vi "frontPanel.vi"(8 "error in (no error)":errorcluster, 10 "closeViewerEvent":refnum<user-event>, 11 "AnalysisResultsViewer in":refnum<class "AnalysisResultsViewer.lvclass">) -> (0 "error out":errorcluster, 3 "AnalysisResultsViewer out":refnum<class "AnalysisResultsViewer.lvclass">)   [LabVIEW 2011, in "Views.lvlib" / "Camera.lvlib" / "AnalysisResultsViewer.lvclass"]
uses:
  AnalysisResultsViewer.lvclass
  AnalysisResultsViewer.lvclass/AnalysisResultsViewer.ctl
panel:
  in  "timescale":dbl=1000.0
  in  "ResultsBox":i32(listbox)
  out "Cloud Size y":dbl(graph)
  in  "stop":bool
  out "Cloud Size x":dbl(graph)
  out "Atom Number":dbl(graph)
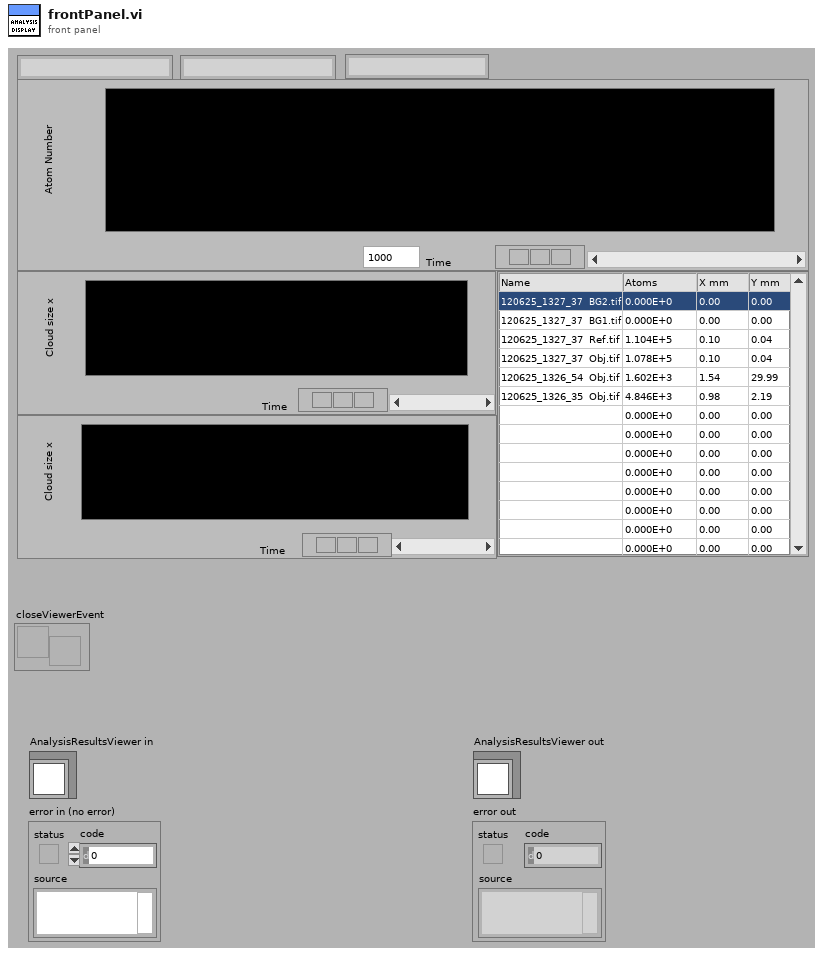
[diagram p1: front panel]
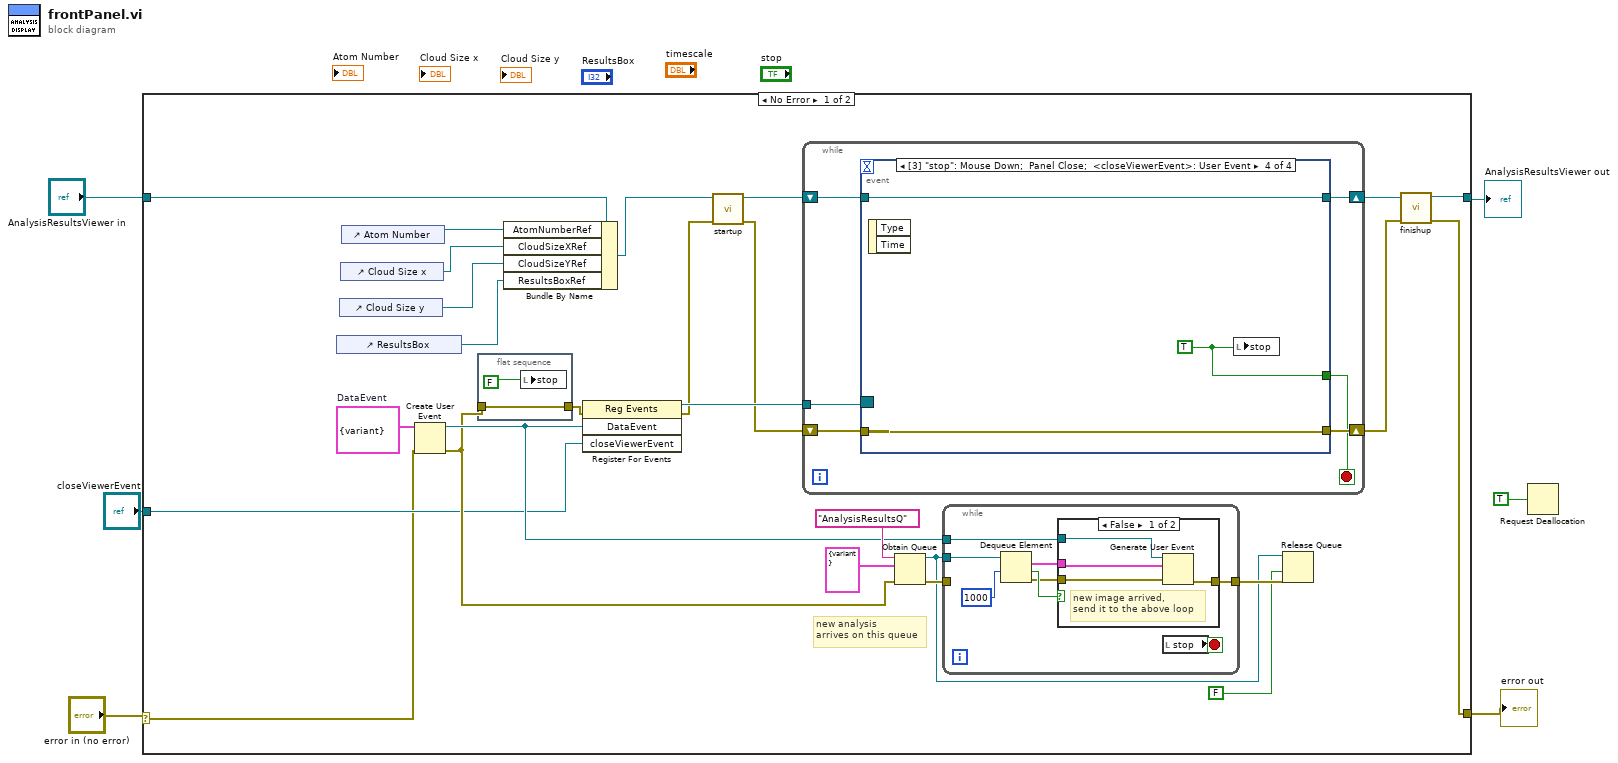
[diagram p0: block diagram]
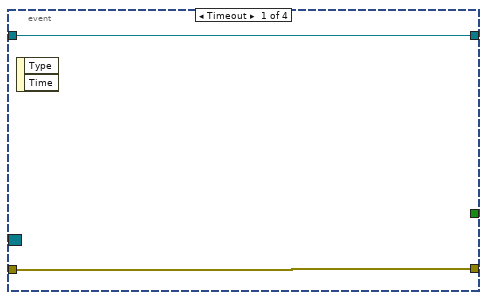
[diagram p3: hidden frame]
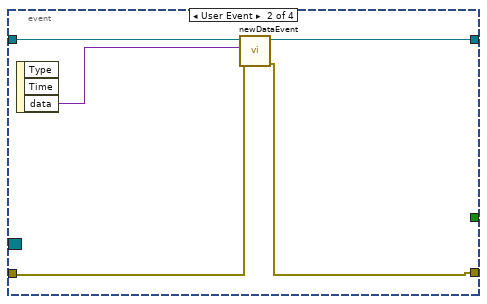
[diagram p4: hidden frame]
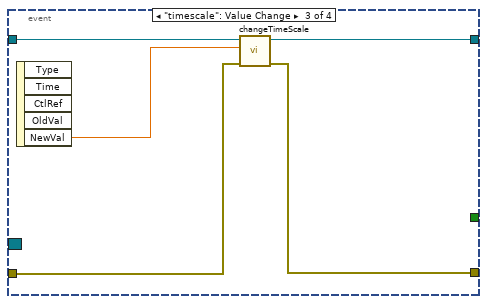
[diagram p5: hidden frame]
diagram:
  n1 = case shown="No Error" "error in (no error)" {
    selector: "error in (no error)" -> [w7 w70]
    tunnel: [w10 w70] -> w5
    tunnel: [w12 w69] -> w3
    tunnel: "AnalysisResultsViewer in" -> [w25 w69]
    tunnel: "closeViewerEvent" -> [w8 _]
    frame No Error {
      w27 = cluster{"data":variant} {"data"=variant}  # DataEvent
      # "new analysis\narrives on this queue"
      n2 = control-ref of="ResultsBox"() -> (w9:refnum<vi>)
      n3 = control-ref of="Cloud Size y"() -> (w22:refnum<vi>)
      n4 = control-ref of="Cloud Size x"() -> (w23:refnum<vi>)
      n5 = control-ref of="Atom Number"() -> (w24:refnum<vi>)
      n6 = Create User Event(user event datatype=w27, error in=w7) -> (user event=w19:refnum<user-event>, error out=w15:errorcluster)
      n7 = flat-sequence {
        tunnel: w15 -> [w34]
        tunnel: [w34] -> w14
        frame #0 {
          n8 = local write "stop"(FALSE) -> ()
        }
      }
      n9 = Bundle By Name(cluster=w25, "AtomNumberRef"=w24, "CloudSizeXRef"=w23, "CloudSizeYRef"=w22, "ResultsBoxRef"=w9) -> (w21:refnum<class "AnalysisResultsViewer.lvclass">)
      n10 = register-events(error in=w14, w19, w8) -> (reference out=w26:refnum<event-registration>, error out=w18:errorcluster)  [unwired: 1 in]
      n11 = call-dynamic "startup.vi"("error in (no error)"=w18, "AnalysisResultsViewer in"=w21) -> ("error out"=w17:errorcluster, "AnalysisResultsViewer out"=w20:refnum<class "AnalysisResultsViewer.lvclass">)  [unwired: 8 in]
      n12 = while {
        shift-right: [w53] -> w13
        shift-left: w20 -> [w52]
        tunnel: w26 -> [w51]
        shift-right: [w49] -> w11
        shift-left: w17 -> [w50]
        stop <- w48 stop-if-true
        n13 = event shown="[3] \"stop\": Mouse Down;  Panel Close;  <closeViewerEvent>: User Event" {
          selector: w51 -> [_ _ _ _]
          dyn-events: _ -> [_ _ _ _]
          timeout: _ -> [_ _ _ _]
          tunnel: [w55 w59 w64 w67] -> w53
          tunnel: w52 -> [w55 w60 w65 w67]
          tunnel: w50 -> [w54 w57 w62 w68]
          tunnel: [w54 w56 w61 w68] -> w49
          tunnel: [_ _ _ w66] -> w48
          event Timeout {
            n14 = event-data() -> ()  [unwired: 1 in, 2 out]
          }
          event User Event {
            n15 = event-data() -> ("data"=w58:variant)  [unwired: 1 in, 2 out]
            n16 = call-dynamic "newDataEvent.vi"("error in (no error)"=w57, "data"=w58, "AnalysisResultsViewer in"=w60) -> ("error out"=w56:errorcluster, "AnalysisResultsViewer out"=w59:refnum<class "AnalysisResultsViewer.lvclass">)  [unwired: 7 in]
          }
          event "timescale": Value Change {
            n17 = event-data() -> ("NewVal"=w63:dbl)  [unwired: 1 in, 4 out]
            n18 = call "changeTimeScale.vi"("error in (no error)"=w62, "timescale"=w63, "AnalysisResultsViewer in"=w65) -> ("error out"=w61:errorcluster, "AnalysisResultsViewer out"=w64:refnum<class "AnalysisResultsViewer.lvclass">)  [unwired: 7 in]
          }
          event "stop": Mouse Down; Panel Close; User Event {
            w66 = TRUE
            n19 = event-data() -> ()  [unwired: 1 in, 2 out]
            n20 = local write "stop"(w66) -> ()
          }
        }
      }
      n21 = Obtain Queue(name (unnamed)="AnalysisResultsQ", element data type=cluster{"data":variant} {"data"=variant} ("dataQ"), error in (no error)=w15) -> (queue out=w29:refnum<queue>, error out=w31:errorcluster)  [unwired: 2 in, 1 out]
      n22 = while {
        tunnel: w19 -> [w38]
        tunnel: w29 -> [w42]
        tunnel: w31 -> [_]
        tunnel: [w37] -> w30
        stop <- w36 stop-if-true
        n23 = Dequeue Element(queue=w42, timeout in ms (-1)=1000) -> (element=w35:cluster{"data":variant}, timed out?=w40:bool, error out=w39:errorcluster)  [unwired: 1 in, 1 out]
        n24 = case shown="False" w40 {
          tunnel: w39 -> [w46 w47]
          tunnel: w38 -> [w43 _]
          tunnel: [w45 w47] -> w37
          tunnel: w35 -> [w44 _]
          frame False {
            # "new image arrived, \nsend it to the above loop"
            n25 = Generate User Event(user event=w43, event data cluster=w44, error in=w46) -> (error out=w45:errorcluster)  [unwired: 1 out]
          }
          frame True {
            # "timeout"
          }
        }
        n26 = local read "stop"() -> (w36:bool)
      }
      n27 = Release Queue(queue=w29, force destroy? (F)=FALSE, error in (no error)=w30) -> ()  [unwired: 3 out]
      n28 = call-dynamic "finishup.vi"("error in (no error)"=w11, "AnalysisResultsViewer in"=w13) -> ("error out"=w10:errorcluster, "AnalysisResultsViewer out"=w12:refnum<class "AnalysisResultsViewer.lvclass">)  [unwired: 8 in]
    }
    frame Error {
    }
  }
  "error out" <- w5
  "AnalysisResultsViewer out" <- w3
  n29 = Request Deallocation(TRUE ("flag")) -> ()
